vi "FABR-Init Stimulus.vi"(0 "Stimulus":T1={"Destination"="", "Rep rate (/sec)"=30.0, "Alternate Polarity"=FALSE, "Duration (ms)"=0.0, "Ramp (ms)"=16.0, "Fs (Hz)"=5.0, "Frame size (s)"=0.0}, 5 "Frequency":dbl[](array[numeric]), 7 "Npts":i32, 11 "error in (no error)":errorcluster) -> (8 "Tones":dbl[][](array[numeric]), 15 "error out":errorcluster)   [LabVIEW 2020]
uses:
  Typedefs/FABR-Stimulus.ctl
  dfa871ce-f627-4f57-9e62-477edc7472d1.vi
  <vilib>/Analysis/NI_AALBase.lvlib
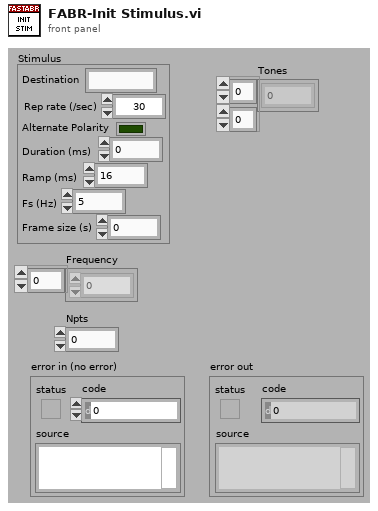
[diagram p1: front panel]
types:
  T1 = typedef "FABR-Stimulus.ctl" = cluster{"Destination":string, "Rep rate (/sec)":dbl, "Alternate Polarity":bool, "Duration (ms)":dbl, "Ramp (ms)":dbl, "Fs (Hz)":dbl, "Frame size (s)":dbl}
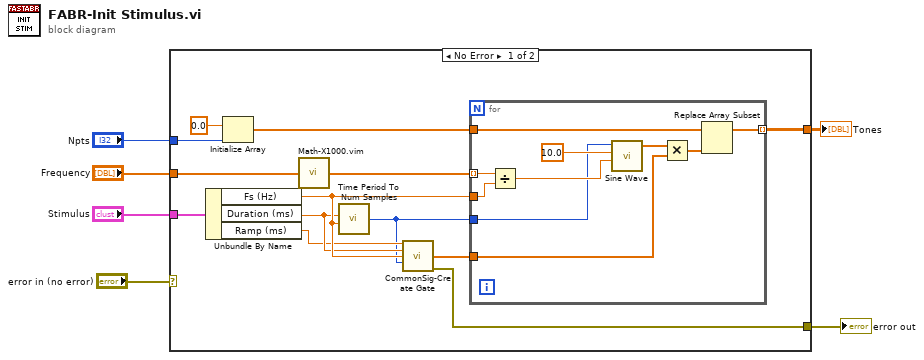
[diagram p0: block diagram]
diagram:
  n1 = case shown="No Error" "error in (no error)" {
    selector: "error in (no error)" -> [_ w30]
    tunnel: "Npts" -> [w19 _]
    tunnel: "Frequency" -> [w16 _]
    tunnel: "Stimulus" -> [w15 _]
    tunnel: [w8 w30] -> w2
    tunnel: [w7 _] -> w1
    frame No Error {
      n2 = Unbundle By Name(w15) -> ("Fs (Hz)"=w13:dbl, "Duration (ms)"=w12:dbl, "Ramp (ms)"=w11:dbl)
      n3 = Initialize Array(0.0, w19) -> (w17:dbl[])
      n4 = call "Math-X1000.vim"("X"=w16) -> ("1000X"=w14:dbl[])
      n5 = call "Time Period To Num Samples.vi"("Duration (ms)"=w12, "Sampling rate (Hz)"=w13) -> ("Samples"=w10:i32)  [unwired: 5 in]
      n6 = call "CommonSig-Create Gate.vi"("Ramp (ms)"=w11, "Duration (ms)"=w12, "Sampling Rate (Hz)"=w13, "Npts"=w10) -> ("Gate"=w9:dbl[], "error out"=w8:errorcluster)  [unwired: 10 in]
      n7 = for {
        tunnel: w17 -> [w22]
        tunnel: w14 -> [w28] mode=indexing
        tunnel: w13 -> [w27]
        tunnel: w10 -> [w25]
        tunnel: w9 -> [w23]
        tunnel: [w20] -> w7 mode=indexing
        n8 = Divide(x=w28, y=w27) -> (x/y=w26:dbl)
        n9 = call <vilib>:"Sine Wave.vi"("samples"=w25, "amplitude"=10.0, "frequency"=w26) -> ("sine wave"=w24:dbl[])  [unwired: 2 in, 2 out]
        n10 = Multiply(x=w24, y=w23) -> (x*y=w21:dbl[])
        n11 = Replace Array Subset(array=w22, new element=w21) -> (w20:dbl[])  [unwired: 1 in]
      }
    }
    frame Error {
    }
  }
  "error out" <- w2
  "Tones" <- w1
